vi "Set pane to its origin.vi"(8 "error in (no error)":errorcluster, 11 "Pane Reference":refnum<vi>) -> (0 "error out (no error)":errorcluster, 3 "Pane Reference out":refnum<vi>)   [LabVIEW 2020]
uses:
  <vilib>/Utility/miscctls.llb/LVPointTypeDef.ctl
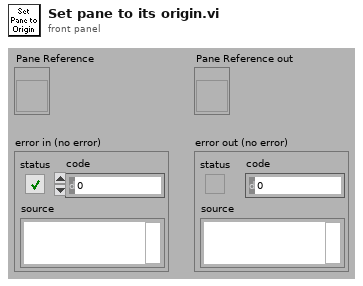
[diagram p1: front panel]
types:
  T1 = typedef "LVPointTypeDef.ctl" = cluster{"Horizontal":i16, "Vertical":i16}
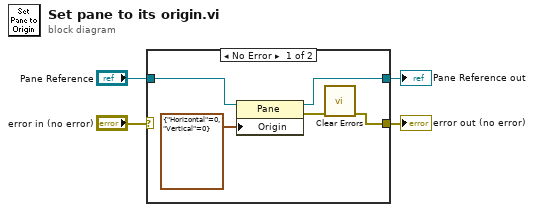
[diagram p0: block diagram]
diagram:
  n1 = case shown="No Error" "error in (no error)" {
    selector: "error in (no error)" -> [_ w11]
    tunnel: "Pane Reference" -> [w9 w10]
    tunnel: [w7 w11] -> w3
    tunnel: [w5 w10] -> w1
    frame No Error {
      n2 = property on="Property Node" class="Pane"(reference=w9, "Origin"=T1 {"Horizontal"=0, "Vertical"=0}) -> (reference out=w5:refnum<vi>, error out=w8:errorcluster)  [unwired: 1 in]
      n3 = call <vilib>:"Clear Errors.vi"("error in (no error)"=w8) -> ("error out"=w7:errorcluster)  [unwired: 5 in, 1 out]
    }
    frame Error {
    }
  }
  "error out (no error)" <- w3
  "Pane Reference out" <- w1
